vi "labview_networktime.vi"() -> ()   [LabVIEW 2018]
panel:
  out "time stamp":timestamp
  out "error out":errorcluster
  in  "stop":bool
  out "port":u16
  out "data out":string
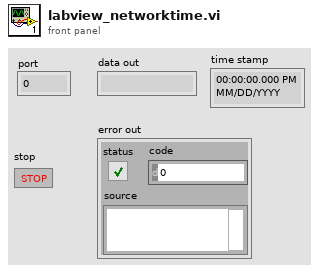
[diagram p1: front panel]
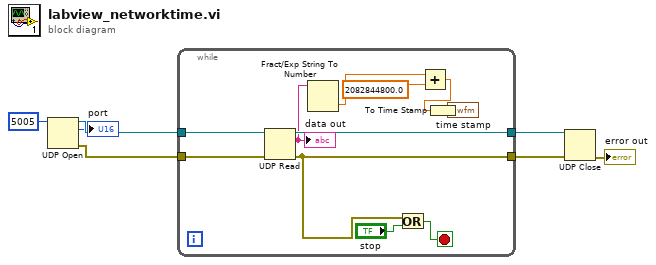
[diagram p0: block diagram]
diagram:
  n1 = UDP Open(11:u16 5005 ("port")) -> (port=w6:refnum<k16>, 0:w3:errorcluster, 2:→"port":u16)  [unwired: 4 in]
  n2 = while {
    tunnel: w6 -> [w18]
    tunnel: [w17] -> w5
    tunnel: [w13] -> w4
    tunnel: w3 -> [w16]
    stop <- w14 stop-if-true
    n3 = UDP Read(connection ID=w18, 8:w16) -> (data out=w12:string, error out=w13:errorcluster, 3:w17:refnum<k16>)  [unwired: 2 in, 2 out]
    "data out" <- w12
    n4 = Fract/Exp String To Number(string=w12) -> (number=w11:dbl)  [unwired: 3 in, 1 out]
    n5 = Or(x=w13, y="stop") -> (x .or. y?=w14:bool)
    n6 = Add(x=w11, y=2082844800.0) -> (x+y=w9:dbl)
    n7 = To Time Stamp(1:w9) -> (0:→"time stamp":timestamp)
  }
  n8 = UDP Close(connection ID=w5, 8:w4) -> (error out=→"error out":errorcluster)  [unwired: 1 out]
